vi "Test.vi"   [LabVIEW 2018, in "Scripts.lvlib"]
uses:
  Scripts.lvlib
  tests/Tests.lvlib
panel:
  # "Overview: Runs all of the tests\nRequirements: LabVIEW\nInstructions: Run this VI."
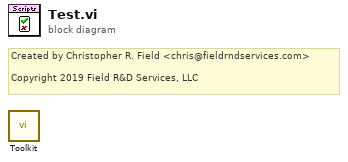
[diagram p0: block diagram]
diagram:
  # "Created by Christopher R. Field <chris@fieldrndservices.com>\n\nCopyright 2019 Field R&D Services, LLC"
  n1 = call "Toolkit.vi"() -> ()  [unwired: 11 in, 1 out]
